vi "PCO_GetImageTransferMode.vi"(8 "error in (no error)":errorcluster {"code" format="%x"}, 11 "ph":u64) -> (0 "error out":errorcluster {"code" format="%x"}, 1 "param":T1, 2 "ErrorMessage":i32 format="%x", 3 "ph out":u64)   [LabVIEW 2019, in "SDK.lvlib" / "SpecialCommandsDimax.lvlib"]
doc: "<b>Description:</b>\nCurrent image transfer mode settings are queried from the camera and the IMAGE_TRANSFER_MODE_PARAM structure is filled with this information.\n\n<b>Supported camera type:</b>\npco.dimax with GigE or USB interface\n\n<b>Descriptor dependency:</b>\nNone"
uses:
  SpecialCommandsDimax.lvlib
  Structures/Structures.lvlib
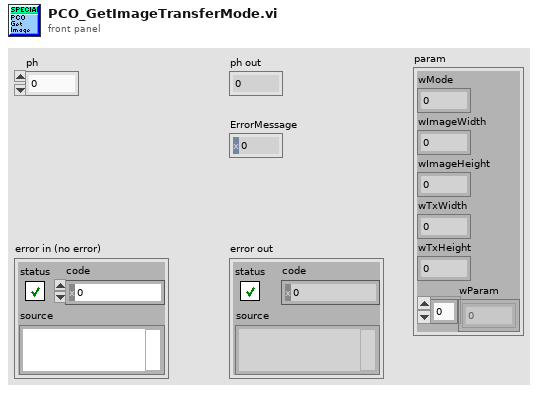
[diagram p1: front panel]
types:
  T1 = cluster{"wMode":u16, "wImageWidth":u16, "wImageHeight":u16, "wTxWidth":u16, "wTxHeight":u16, "wParam":u16[]}
  T2 = cluster{"wSize":u16, "wMode":u16, "wImageWidth":u16, "wImageHeight":u16, "wTxWidth":u16, "wTxHeight":u16, "wParam":cluster{u16, u16, u16, u16, u16, u16, u16, u16}, "ZZwDummy":cluster{u16, u16, u16, u16, u16, u16, u16, u16, u16, u16}}
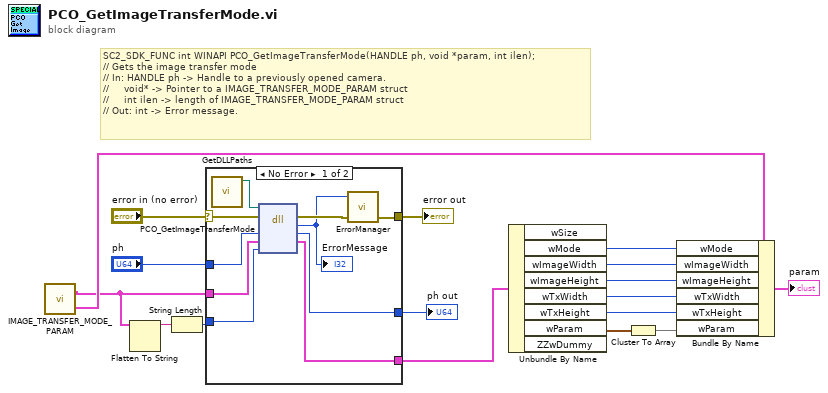
[diagram p0: block diagram]
diagram:
  # "SC2_SDK_FUNC int WINAPI PCO_GetImageTransferMode(HANDLE ph, void *param, int ilen);\n// Gets the image transfer mode\n// In: HANDLE ph -> Handle to a previously opened camera.\n//     void* -> Pointer to a IMAGE_TRANSFER_MODE_PARAM struct\n//     int ilen -> length of IMAGE_TRANSFER_MODE_PARAM struct\n// Out: int -> Error message."
  n1 = call "IMAGE_TRANSFER_MODE_PARAM.vi"() -> ("IMAGE_TRANSFER_MODE_PARAM"=w12:T1, "IMAGE_TRANSFER_MODE_PARAM_RAW"=w2:T2)  [unwired: 4 in, 2 out]
  n2 = Flatten To String(anything=w2) -> (data string=w3:string)  [unwired: 3 in, 2 out]
  n3 = String Length(string=w3) -> (length=w1:i32)
  n4 = case shown="No Error" "error in (no error)" {
    selector: "error in (no error)" -> [w22 w28]
    tunnel: "ph" -> [w27 w30]
    tunnel: [w26 w30] -> w16
    tunnel: w2 -> [w25 w29]
    tunnel: [w24 w29] -> w13
    tunnel: w1 -> [w23 _]
    tunnel: [w20 w28] -> w15
    frame No Error {
      n5 = call "GetDLLPaths.vi"() -> ("SC2_Cam_Path"=w18:path)  [unwired: 8 in, 3 out]
      n6 = dll-call lib="?" fn="PCO_GetImageTransferMode"(path in=w18, error in=w22, "ph"=w27, "param"=w25, "ilen"=w23) -> (error out=w21:errorcluster, "return type"=w19:i32, "ph"=w26:u64, "param"=w24:T2)  [unwired: 2 in, 1 out]
      "ErrorMessage" <- w19
      n7 = call "ErrorManager.vi"("error in (no error)"=w21, "error code"=w19) -> ("error out"=w20:errorcluster)  [unwired: 2 in, 1 out]
    }
    frame Error {
    }
  }
  "ph out" <- w16
  "error out" <- w15
  n8 = Unbundle By Name(w13) -> ("wMode"=w11:u16, "wImageWidth"=w10:u16, "wImageHeight"=w9:u16, "wTxWidth"=w8:u16, "wTxHeight"=w7:u16, "wParam"=w6:cluster{u16, u16, u16, u16, u16, u16, u16, u16})  [unwired: 2 out]
  n9 = Cluster To Array(cluster=w6) -> (array=w5:u16[])
  n10 = Bundle By Name(cluster=w12, "wMode"=w11, "wImageWidth"=w10, "wImageHeight"=w9, "wTxWidth"=w8, "wTxHeight"=w7, "wParam"=w5) -> (→"param":T1)
